vi "Inject Some Thangs.vi"(8 "error in (no error)":errorcluster, 9 "Attributes Ref":refnum<data-value>, 11 "iTest Step in":refnum<class "iTest Step.lvclass">) -> (0 "error out":errorcluster, 3 "iTest Step out":refnum<class "iTest Step.lvclass">)   [LabVIEW 2017, in "Parallelizer Example.lvlib" / "iTest Step.lvclass"]
uses:
  <vilib>/gpm_packages/@cs/test-executive/Source/Sandbox/Parallelizer Example/iTest Step/iTest Step.lvclass
  <vilib>/gpm_packages/@cs/lookup-table/Source/LookupTable/LookupTable.lvclass
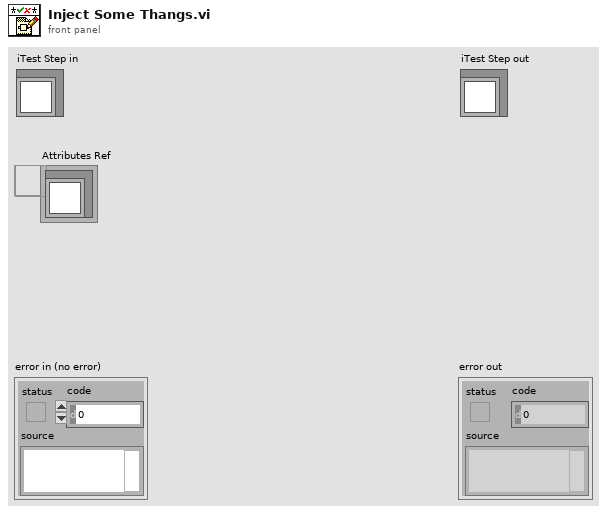
[diagram p1: front panel]
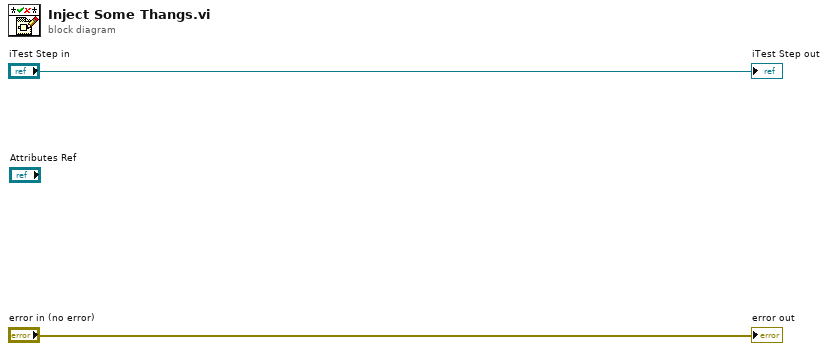
[diagram p0: block diagram]
diagram:
  "error out" <- "error in (no error)"
  "iTest Step out" <- "iTest Step in"
